vi "7.7-Reliable UPD Client Template.vi"() -> ()   [LabVIEW 2010]
doc: "This VI implements a client for the Named Service UDP Server.vi.\nIt connects to a service by specifying the server address and the name of the service. After sending a 'Hello' string to the server, the client receives the string sent by the server, displays the string and closes the connection.\n\n<b>Note:</b> This VI is built to work with the Named Service UDP Server.vi in UDP.llb.\nUDP Mutlicast Addressing Scheme:\n\n3.7 - Multicast Address: 224.0.3.7\n3.1-4.7.1 Port: 31471\n3.2-4.7.2 Port: 32472\n3.3-4.7.3 Port: 33473\n3.4-4.7.4 Port: 34474\n\n5.7 - Multicast Address: 224.0.5.7\n5.1-4.7.1 Port: 51471\n5.2-4.7.2 Port: 52472\n5.3-4.7.3 Port: 53473\n5.4-4.7.4 Port: 54474\n\n5.1-6.7.1 Port: 51671\n5.2-6.7.2 Port: 52672\n5.3-6.7.3 Port: 53673\n5.4-6.7.4 Port: 54674\n\n7.7 - Multicast Address: 224.0.7.7\n7.1-6.7.1 Port: 61671\n7.2-6.7.2 Port: 62672\n7.3-6.7.3 Port: 63673\n7.4-6.7.4 Port: 64674"
uses:
  4-High Neurons/4.0-Timing Badass.ctl
  6-OCU Neurons/6.4-How Reporting Typedef.ctl
  <vilib>/Utility/tcp.llb/UDP Multicast Open.vi
  7.0-Global.vi
  5-Forebrain/5.7-UDP/5.7-UDP Check Checksum.vi
  <vilib>/addons/internet/NI_InternetTK_Common_VIs.lvlib
panel:
  out "data":T1
  out "Super Heart Beat":T2
  out "Error":errorcluster
  in  "stop":bool
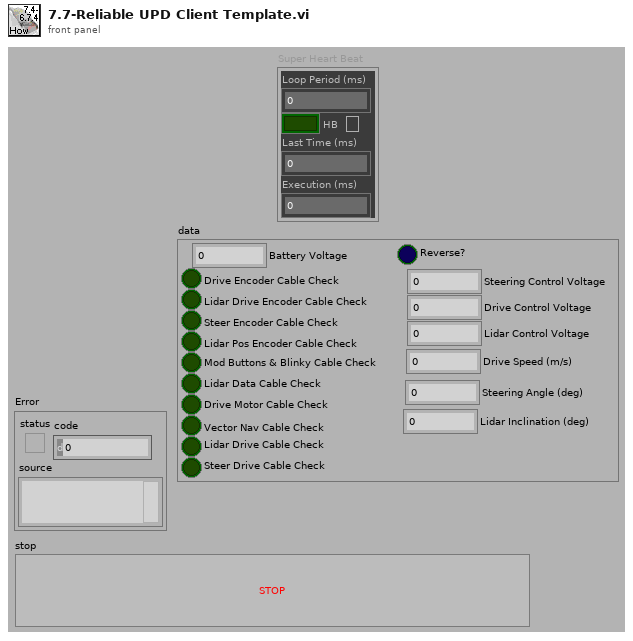
[diagram p1: front panel]
types:
  T1 = typedef "6.4-How Reporting Typedef.ctl" = cluster{"Drive Speed (m/s)":dbl, "Lidar Inclination (deg) ":dbl, "Steering Angle (deg)":dbl, "Battery Voltage":dbl, "Drive Encoder Cable Check":bool, "Lidar Drive Encoder Cable Check":bool, "Steer Encoder Cable Check":bool, "Lidar Pos Encoder Cable Check":bool, "Mod Buttons & Blinky Cable Check":bool, "Lidar Data Cable Check":bool, "Drive Motor Cable Check":bool, "Vector Nav Cable Check":bool, "Lidar Drive Cable Check":bool, "Steer Drive Cable Check":bool, "Reverse?":bool, "Steering Control Voltage":dbl, "Drive Control Voltage":dbl, "Lidar Control Voltage":dbl}
  T2 = typedef "4.0-Timing Badass.ctl" = cluster{"Loop Period (ms)":u32, "HB":bool, "Last Time (ms)":u32, "Execution (ms)":u32}
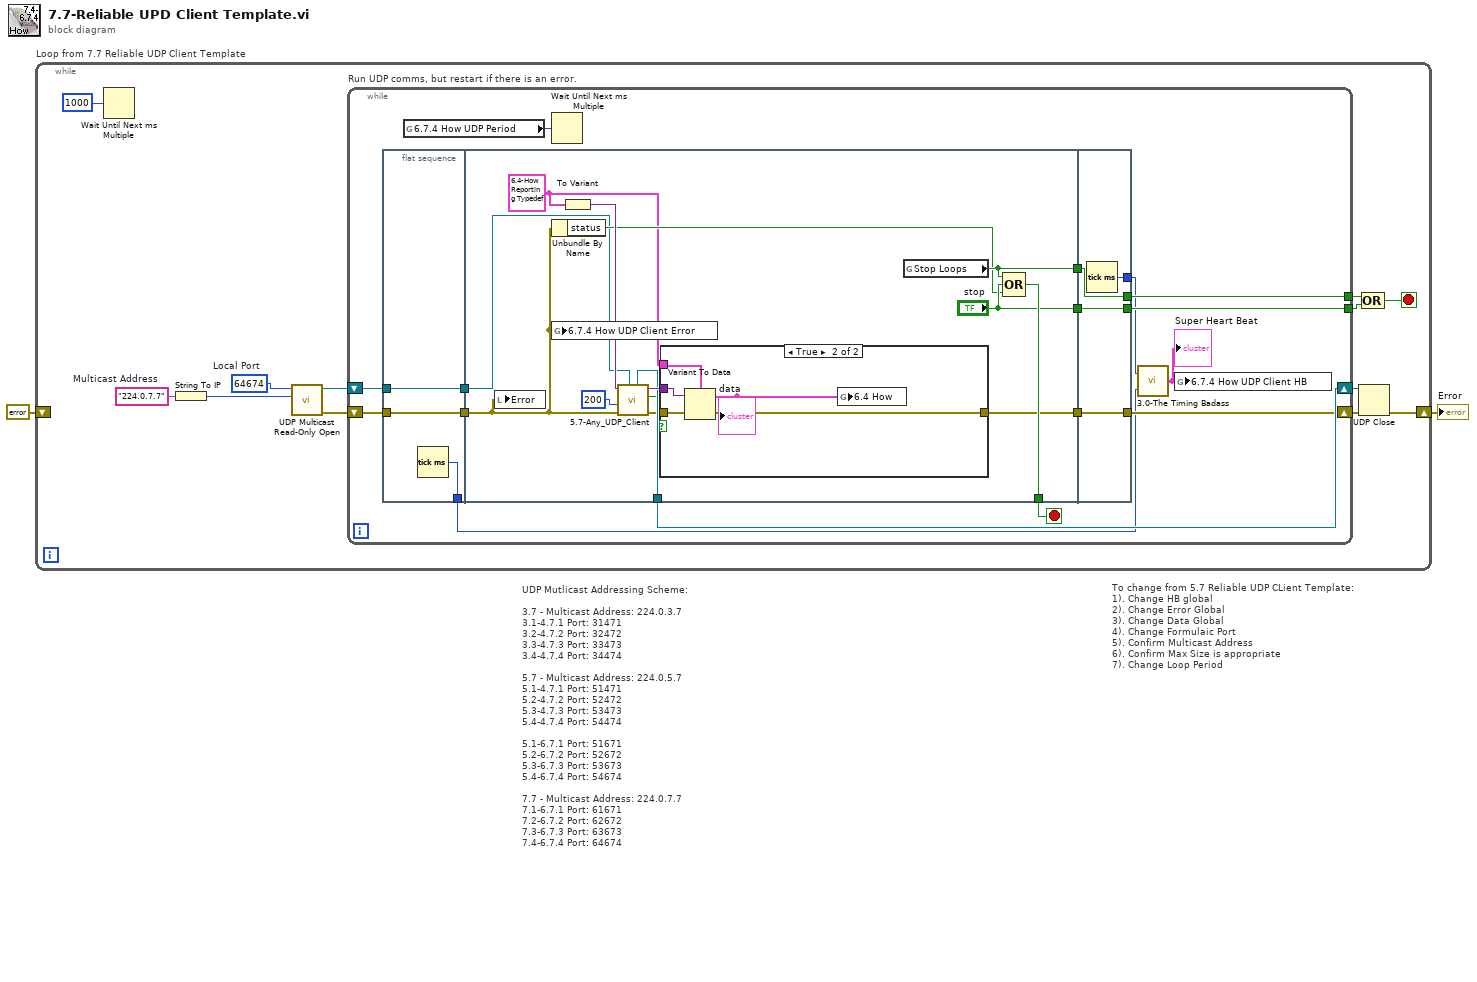
[diagram p0: block diagram]
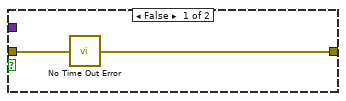
[diagram p2: hidden frame]
diagram:
  # "To change from 5.7 Reliable UDP CLient Template:\n1). Change HB global\n2). Change Error Global\n3). Change Data Global\n4). Change Formulaic Port\n5). Confirm Multicast Address\n6). Confirm Max Size is appropriate\n7). Change Loop Period"
  # "UDP Mutlicast Addressing Scheme:\n\n3.7 - Multicast Address: 224.0.3.7\n3.1-4.7.1 Port: 31471\n3.2-4.7.2 Port: 32472\n3.3-4.7.3 Port: 33473\n3.4-4.7.4 Port: 34474\n\n5.7 - Multicast Address: 224.0.5.7\n5.1-4.7.1 Port: 51471\n5.2-4.7.2 Port: 52472\n5.3-4.7.3 Port: 53473\n5.4-4.7.4 Port: 54474\n\n5.1-6.7.1 Port: 51671\n5.2-6.7.2 Port: 52672\n5.3-6.7.3 Port: 53673\n5.4-6.7.4 Port: 54674\n\n7.7 - Multicast Address: 224.0.7.7\n7.1-6.7.1 Port: 61671\n7.2-6.7.2 Port: 62672\n7.3-6.7.3 Port: 63673\n7.4-6.7.4 Port: 64674"
  n1 = while "Loop from 7.7 Reliable UDP Client Template" {
    shift-right: [w9] -> w2
    shift-left: errorcluster {"status"=FALSE, "code"=0, "source"=""} ("error out") -> [_]
    stop <- w12 stop-if-true
    w5 = u16 64674  # Local Port
    w7 = "224.0.7.7"  # Multicast Address
    n2 = Wait Until Next ms Multiple(millisecond multiple=u32 1000) -> ()  [unwired: 1 out]
    n3 = String To IP(1:w7) -> (0:w6:u32)
    n4 = call-poly <vilib>:"UDP Multicast Read-Only Open.vi"("multicast addr"=w6, "port"=w5) -> ("error out"=w3:errorcluster, "connection ID"=w4:refnum<k16>)  [unwired: 2 in, 6 out]
    n5 = while "Run UDP comms, but restart if there is an error." {
      tunnel: [w29] -> w14
      tunnel: [w28] -> w13
      shift-right: [w26] -> w11
      shift-left: w4 -> [w27]
      shift-right: [w25] -> w10
      shift-left: w3 -> [w24]
      stop <- w30 stop-if-true
      n6 = flat-sequence {
        tunnel: w24 -> [w32]
        tunnel: w27 -> [w33]
        tunnel: [w33] -> w22
        tunnel: [w32] -> w21
        tunnel: [w31] -> w16
        tunnel: [w47] -> w30
        tunnel: [w40] -> w26
        tunnel: w22 -> [w41]
        tunnel: w21 -> [w36]
        tunnel: [w44] -> w20
        tunnel: ["stop"] -> w19
        tunnel: [w39] -> w18
        tunnel: [w56] -> w25
        tunnel: [w57] -> w28
        tunnel: [w58] -> w29
        tunnel: w20 -> [w58]
        tunnel: w19 -> [w57]
        tunnel: w18 -> [w56]
        tunnel: [w55] -> w17
        frame #0 {
          n7 = Tick Count (ms)() -> (millisecond timer value=w31:u32)
        }
        frame #1 {
          w34 = T1 {"Drive Speed (m/s)"=0.0, "Lidar Inclination (deg) "=0.0, "Steering Angle (deg)"=0.0, "Battery Voltage"=0.0, "Drive Encoder Cable Check"=FALSE, "Lidar Drive Encoder Cable Check"=FALSE, "Steer Encoder Cable Check"=FALSE, "Lidar Pos Encoder Cable Check"=FALSE, "Mod Buttons & Blinky Cable Check"=FALSE, "Lidar Data Cable Check"=FALSE, "Drive Motor Cable Check"=FALSE, "Vector Nav Cable Check"=FALSE, "Lidar Drive Cable Check"=FALSE, "Steer Drive Cable Check"=FALSE, "Reverse?"=FALSE, "Steering Control Voltage"=0.0, "Drive Control Voltage"=0.0, "Lidar Control Voltage"=0.0} ("data")
          n8 = local write "Error"(w36) -> ()
          n9 = Unbundle By Name(w36) -> ("status"=w42:bool)
          n10 = global write "7.0-Global.vi" "6.7.4 How UDP Client Error"(w36) -> ()
          n11 = To Variant(anything=w34) -> (Variant=w46:variant)
          n12 = call "5.7-Any_UDP_Client.vi"("Port In"=w41, "error In"=w36, "Max Size"=200, "DataTypeIn"=w46) -> ("Error Out"=w38:errorcluster, "Check Passed"=w37:bool, "DataOut"=w45:variant, "Port out"=w40:refnum<k16>)  [unwired: 4 in]
          n13 = case "Ignore Timeouts" shown="True" w37 {
            tunnel: w45 -> [_ w54]
            tunnel: w34 -> [_ w53]
            tunnel: w38 -> [w49 w52]
            tunnel: [w48 w51] -> w39
            frame False {
              n14 = call <vilib>:"No Time Out Error.vi"("error in (no error)"=w49) -> ("error out"=w48:errorcluster)  [unwired: 14 in]
            }
            frame True {
              n15 = Variant To Data(error in=w52, Variant=w54, type=w53) -> (error out=w51:errorcluster, data=w50:T1)
              "data" <- w50
              n16 = global write "7.0-Global.vi" "6.4 How"(w50) -> ()
            }
          }
          n17 = global read "7.0-Global.vi" "Stop Loops"() -> (w44:bool)
          n18 = Compound Arithmetic op=OR(w44, "stop", w42) -> (w47:bool)
        }
        frame #2 {
          n19 = Tick Count (ms)() -> (millisecond timer value=w55:u32)
        }
      }
      n20 = global read "7.0-Global.vi" "6.7.4 How UDP Period"() -> (w23:u32)
      n21 = Wait Until Next ms Multiple(millisecond multiple=w23) -> ()  [unwired: 1 out]
      n22 = call "3.0-The Timing Badass.vi"("Start"=w16, "End"=w17) -> ("Super Heart Beat"=w15:T2)
      "Super Heart Beat" <- w15
      n23 = global write "7.0-Global.vi" "6.7.4 How UDP Client HB"(w15) -> ()
    }
    n24 = UDP Close(connection ID=w11, 8:w10) -> (error out=w9:errorcluster)  [unwired: 1 out]
    n25 = Compound Arithmetic op=OR(w14, w13) -> (w12:bool)
  }
  "Error" <- w2
